vi "DFD MRate Filtering for Single Block.vi"   [LabVIEW 2017, in "NI_DigFilterLicensed.lvlib"]
doc: "Filters a single-block signal with a multirate filter. Wire data to the <B>signal in</B> input to determine the polymorphic instance to use or manually select the instance."
uses:
  <vilib>/addons/Digital Filter Design/NI_DigFilterLicensed.lvlib
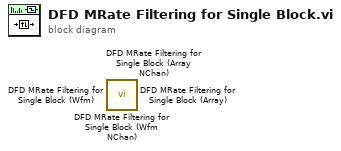
[diagram p0: block diagram]
diagram:
  n1 = call <vilib>:"DFD MRate Filtering for Single Block (Wfm NChan).vi"() -> ()  [unwired: 10 in, 2 out]
  n2 = call <vilib>:"DFD MRate Filtering for Single Block (Array NChan).vi"() -> ()  [unwired: 10 in, 2 out]
  n3 = call <vilib>:"DFD MRate Filtering for Single Block (Wfm).vi"() -> ()  [unwired: 10 in, 2 out]
  n4 = call <vilib>:"DFD MRate Filtering for Single Block (Array).vi"() -> ()  [unwired: 10 in, 2 out]
